vi "Measure Voltage Waveform.vi"(0 "Scope Reference":refnum<k15>, 5 "Scope Channels":string, 7 "Record Length":dbl, 9 "Actual Sample Rate":dbl, 11 "error in (no error)":errorcluster) -> (4 "Input Waveform":T1, 6 "Output Waveform":T1, 15 "error out":errorcluster)   [LabVIEW 2020, in "LDO PSRR.lvlib"]
uses:
  LDO PSRR.lvlib
  <instrlib>/niScope/Acquire/Fetch/niScope Multi Fetch Cluster.vi
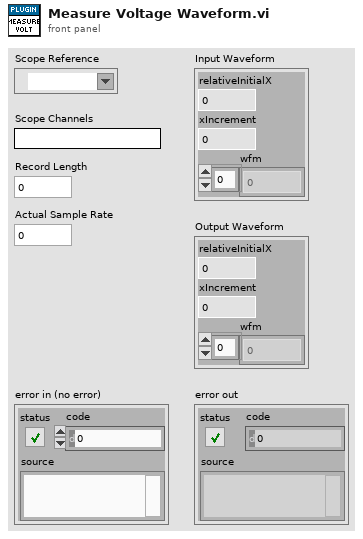
[diagram p1: front panel]
types:
  T1 = cluster{"relativeInitialX":dbl, "xIncrement":dbl, "wfm":dbl[]}
  T2 = cluster{"relativeInitialX":dbl, "xIncrement":dbl, "wfm":dbl[]}[]
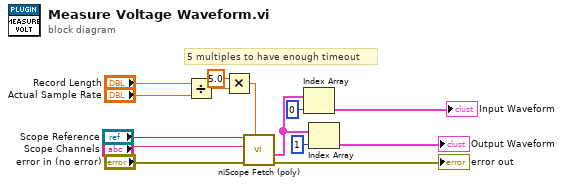
[diagram p0: block diagram]
diagram:
  # "5 multiples to have enough timeout"
  n1 = Divide(x="Record Length", y="Actual Sample Rate") -> (x/y=w6:dbl)
  n2 = Multiply(x=5.0, y=w6) -> (x*y=w10:dbl)
  n3 = call-poly <instrlib>:"niScope Fetch (poly).vi"("timeout"=w10, "error in"="error in (no error)", "channels"="Scope Channels", "instrument handle"="Scope Reference") -> ("error out"=→"error out":errorcluster, "waveform"=w5:T2)  [unwired: 4 in, 2 out]
  n4 = Index Array(array=w5, index=0) -> (element=→"Input Waveform":T1)
  n5 = Index Array(array=w5, index=1) -> (element=→"Output Waveform":T1)
